vi "Log_open_or_create_file.vi"(10 "Data file name:":path, 11 "File header":string) -> ()   [LabVIEW 2018]
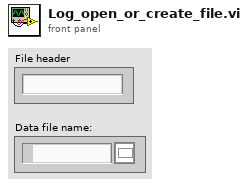
[diagram p1: front panel]
types:
  T1 = enum16{"open", "replace", "create", "open or create", "replace or create", "replace or create with confirmation"}
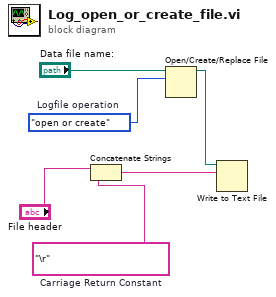
[diagram p0: block diagram]
diagram:
  w4 = "\r"  # Carriage Return Constant
  w5 = T1."open or create"  # Logfile operation
  n1 = Concatenate Strings "Concatenate Strings"("File header", w4) -> (w2:string)
  n2 = Open/Create/Replace File(file path (use dialog)="Data file name:", operation (0:open)=w5) -> (refnum out=w3:refnum<file>)  [unwired: 4 in, 2 out]
  n3 = Write to Text File(file (use dialog)=w3, text=w2) -> ()  [unwired: 2 in, 3 out]
